vi "StrToWave.vi"(11 "String":string) -> (3 "Data":cluster{u16, u16})   [LabVIEW 2017]
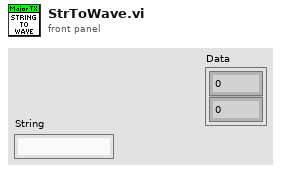
[diagram p1: front panel]
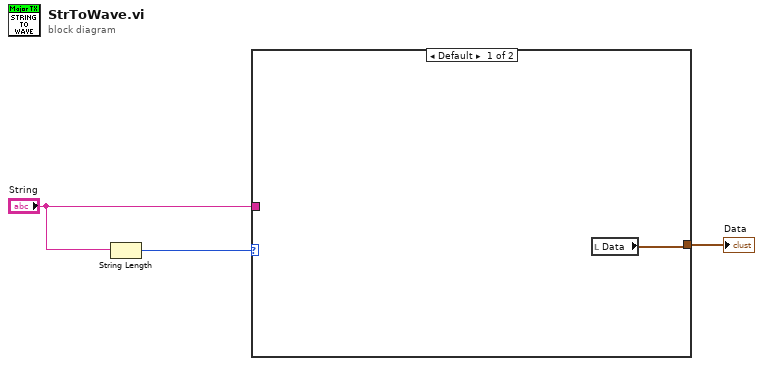
[diagram p0: block diagram]
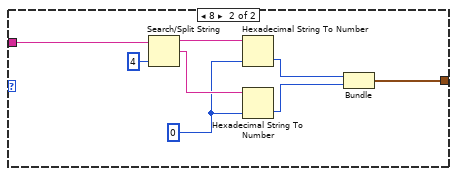
[diagram p2: hidden frame]
diagram:
  n1 = String Length(string="String") -> (length=w2:i32)
  n2 = case shown="Default" w2 {
    tunnel: "String" -> [_ w6]
    tunnel: [w4 w5] -> w1
    frame Default {
      n3 = local read "Data"() -> (w4:cluster{u16, u16})
    }
    frame 8 {
      w10 = u16 0 ("default (0 U32)")
      n4 = Search/Split String(string=w6, offset (0)=4) -> (substring before match=w12:string, match + rest of string=w11:string)  [unwired: 1 in, 1 out]
      n5 = Hexadecimal String To Number(string=w12, default (0uL)=w10) -> (number=w9:u16)  [unwired: 1 in, 1 out]
      n6 = Hexadecimal String To Number(string=w11, default (0uL)=w10) -> (number=w8:u16)  [unwired: 1 in, 1 out]
      n7 = Bundle(w9, w8) -> (w5:cluster{u16, u16})  [unwired: 1 in]
    }
  }
  "Data" <- w1
